vi "Test No Private Methods Found.vi"(11 "Test Case In":refnum<class "Test Method Finding Test.lvclass">) -> (0 "error out":errorcluster, 3 "Test Case Out":refnum<class "Test Method Finding Test.lvclass">)   [LabVIEW 2020, in "Test Method Finding Test.lvclass"]
uses:
  Test Method Finding Test.lvclass
  C:/Program Files (x86)/National Instruments/LabVIEW 2020/vi.lib/Astemes/LUnit/Test Case.lvclass
  Test Doubles/Test Case Test Double/Test Case Test Double.lvclass
  <vilib>/Astemes/LUnit/Test Case.lvclass/Test Case.ctl
  94179ef5-e4c8-4fab-b65e-e568f62fadc2.vi
  <vilib>/Astemes/LUnit/Palette/Fail If.vi
  <vilib>/Astemes/LUnit/Core/LUnit Test Case/Private/Append Pass Result.vi
  <vilib>/Astemes/LUnit/Core/LUnit Test Case/Private/Append Fail Result.vi
  <vilib>/Astemes/LUnit/Core/LUnit Test Case/Private/Run In UI.vi
  <vilib>/Utility/error.llb/Clear Errors.vi
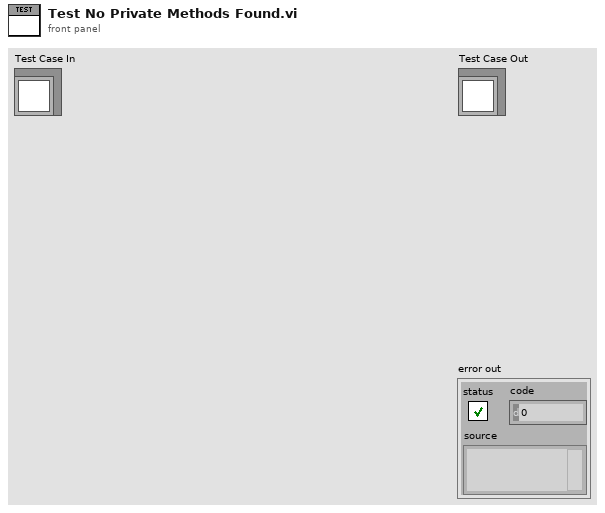
[diagram p1: front panel]
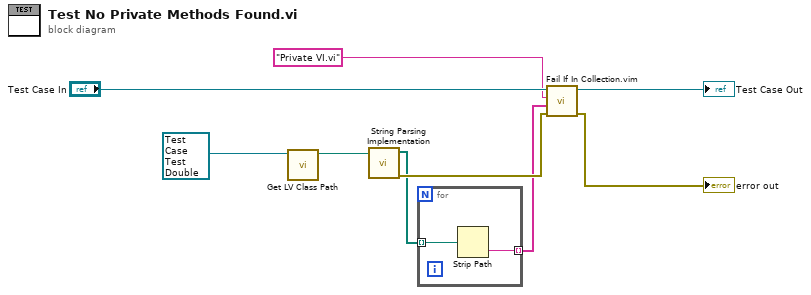
[diagram p0: block diagram]
diagram:
  n1 = call <vilib>:"Get LV Class Path.vi"("object"=refnum<class "Test Case Test Double.lvclass"> refnum ("Test Case Test Double.lvclass")) -> ("class path"=w4:path)  [unwired: 9 in, 1 out]
  n2 = call "String Parsing Implementation.vi"("class path"=w4) -> ("error out"=w6:errorcluster, "Array"=w2:path[])  [unwired: 9 in]
  n3 = for {
    tunnel: w2 -> [w11] mode=indexing
    tunnel: [w10] -> w1 mode=indexing
    n4 = Strip Path(path=w11) -> (name=w10:string)  [unwired: 1 out]
  }
  n5 = call "Fail If In Collection.vim"("error in (no error)"=w6, "Collection"=w1, "Element"="Private VI.vi" ("Array"), "LUnit Test Case In"="Test Case In") -> ("error out"=→"error out":errorcluster, "LUnit Test Case Out"=→"Test Case Out":refnum<class "Test Method Finding Test.lvclass">)  [unwired: 6 in]
